vi "THz AcqPan.vi"(8 "error in (no error)":errorcluster caption="entrée d'erreur (pas d'erreur)", 11 "SR830.lvclass":refnum<class "SR830.lvclass">) -> (0 "error out":errorcluster caption="sortie d'erreur", 3 "SR830.lvclass Out":refnum<class "SR830.lvclass">)   [LabVIEW 2012, in "SR830.lvclass"]
uses:
  SR830.lvclass
  BaseDevice/Accessor/GetClassEvent.vi
panel:
  in  "On/Off Delay(ms)":dbl min=0.0 max=10000.0 step=1.0
  in  "Shutter":bool
  out "Sensitivity":u16(ring)=1 items=["2 nV/fA", "5 nV/fA", "10 nV/fA", "20 nV/fA", "50 nV/fA", "100 nV/fA", "200 nV/fA", "500 nV/fA", "1 µV/pA", "2 µV/pA", "5 µV/pA", "10 µV/pA", "20 µV/pA", "50 µV/pA", "100µV/pA", "200 µV/pA", "500µV/pA", "1 mV/nA", "2 mV/nA", "5 mV/nA", "10 mV/nA", "20 mV/nA", "50 mV/nA", "100 mV/nA", "200 mV/nA", "500 mV/nA", "1 V/uA"]
  in  "Acq":bool
  out "Phase":dbl=1000.0 caption="Phase (°)" min=0.0 step=0.1 format="%#_5f"
  out "MAG":dbl=1000.0 caption="MAG (V)" min=0.0 step=0.1 format="%^#_6e"
  out "UNLCK":bool caption="SpexMov"
  out "X":dbl=1000.0 caption="X (V)" min=0.0 step=0.1 format="%^#_6e"
  in  "Stop":bool
  out "Init Program":bool
  out "OVLD":bool caption="SpexMov"
  in  "Update":bool caption="stopSpectro"
  out "Y":dbl=1000.0 caption="Y (V)" min=0.0 step=0.1 format="%^#_6e"
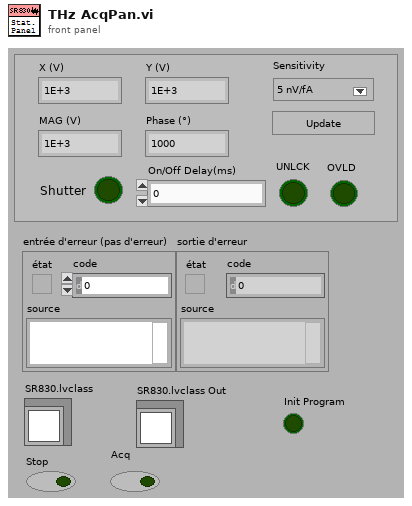
[diagram p1: front panel]
types:
  T1 = enum8{"Enabled", "Disabled", "Disabled and Grayed Out"}
  T2 = enum16{"Phase Shift", "Reference Source", "Reference Frequency", "Reference Trigger", "Detection Harmonic", "Sine Amplitude", "Input Configuration", "Input Shield", "Input Coupling", "Input Line Notch Filter", "Sensitivity", "Dynamic Reserve", "Time Constant", "Low Pass Filter", "Sync Filter", "Expand X", "Expand Y", "Expand R", "All"}
  T3 = cluster{"Phase Shift (°)":dbl, "Reference Source":u16, "Frequency (Hz)":dbl, "Reference Trigger":u16, "Harmonic":i32, "Sine Amplitude (V)":dbl, "Input Configuration":u16, "Input Shield":u16, "Input Coupling":u16, "Input Notch Filters":cluster{"1xLineFilter":bool, "2xLineFilter":bool}, "Sensitivity":u16, "Dynamic Reserve":u16, "Time Constant":u16, "Low Pass Filter":u16, "Sync Filter":bool, "Expand X":cluster{"Offset (%)":dbl, "Expand":u16}, "Expand Y":cluster{"Offset (%)":dbl, "Expand":u16}, "Expand R":cluster{"Offset (%)":dbl, "Expand":u16}}
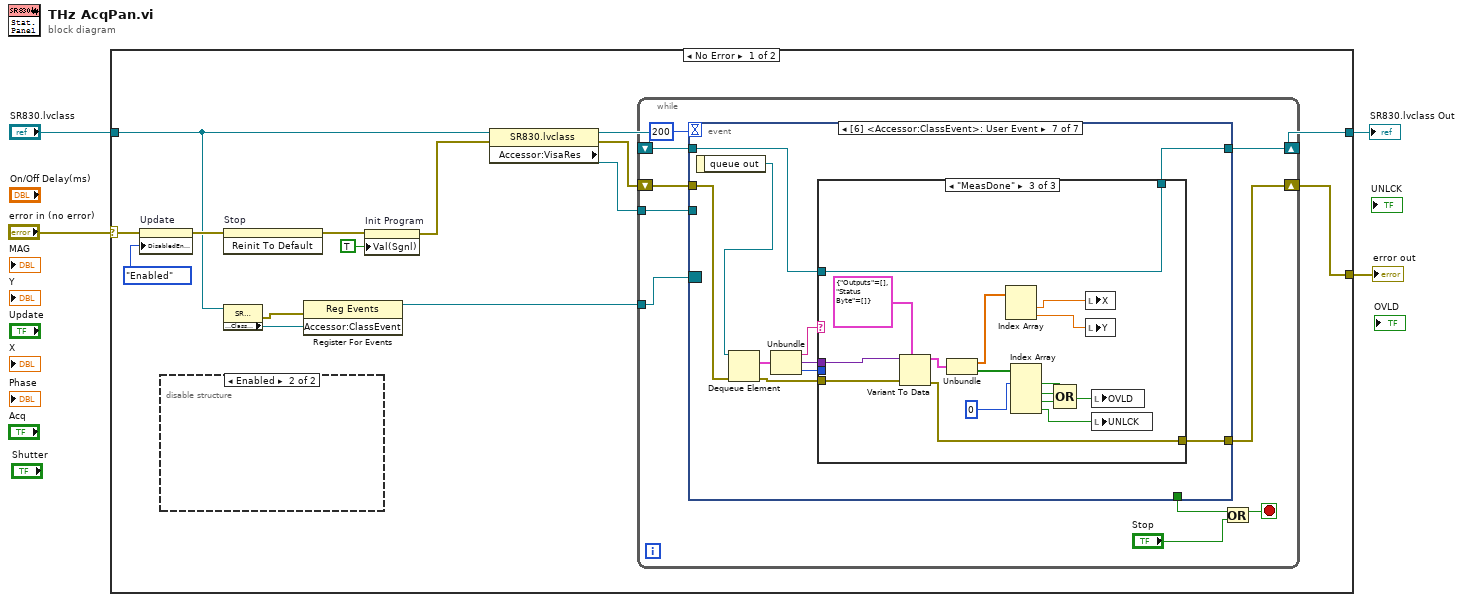
[diagram p0: block diagram]
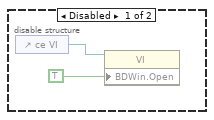
[diagram p2: hidden frame]
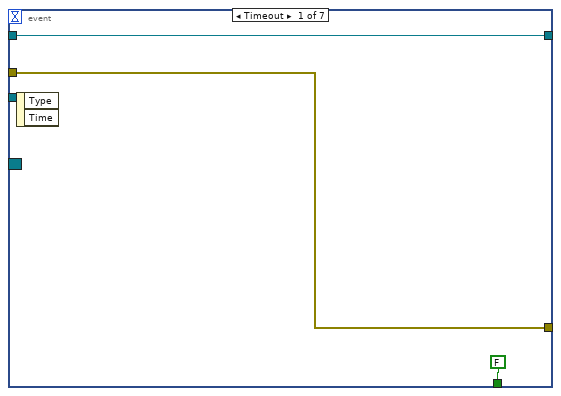
[diagram p3: hidden frame]
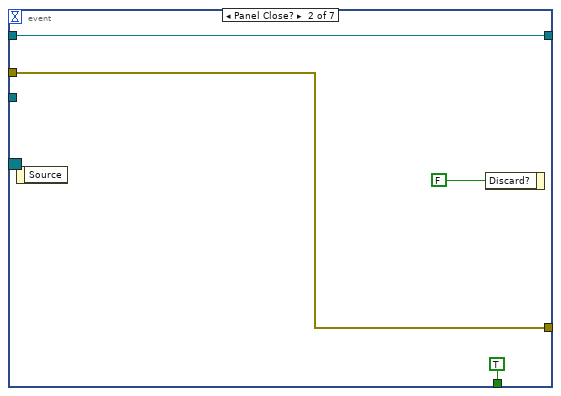
[diagram p4: hidden frame]
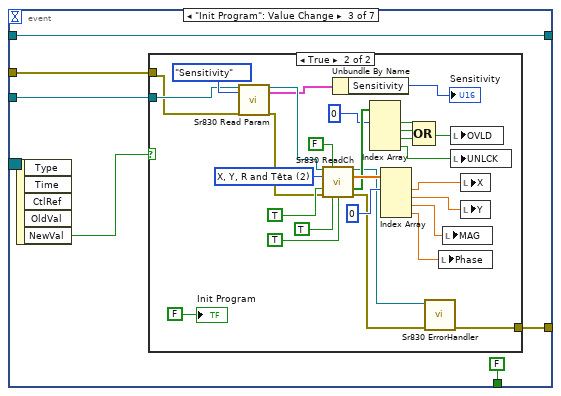
[diagram p5: hidden frame]
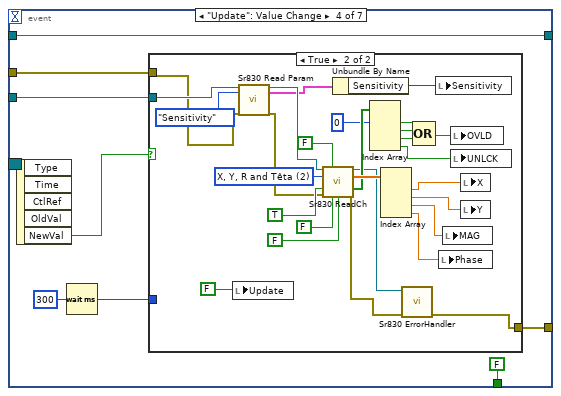
[diagram p7: hidden frame]
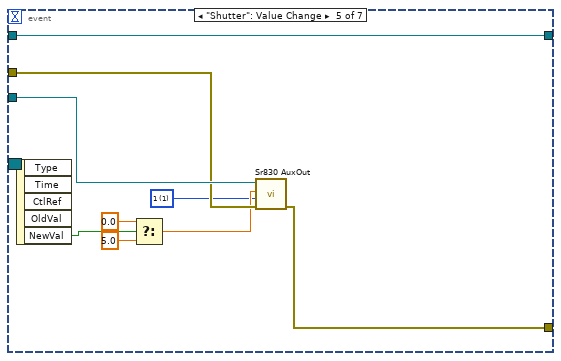
[diagram p9: hidden frame]
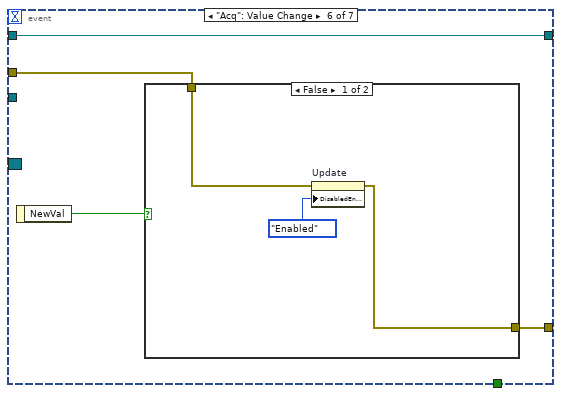
[diagram p10: hidden frame]
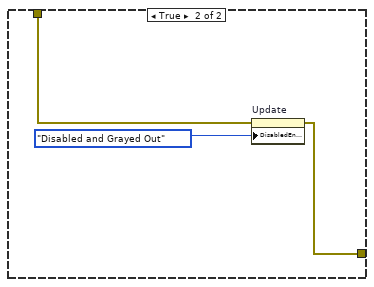
[diagram p11: hidden frame]
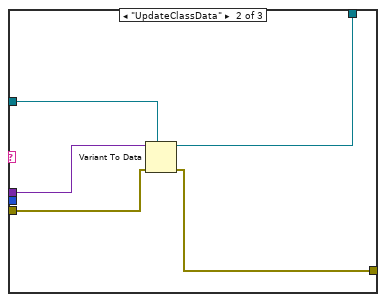
[diagram p13: hidden frame]
diagram:
  n1 = case shown="No Error" "error in (no error)" {
    selector: "error in (no error)" -> [w11 w165]
    tunnel: [w5 w165] -> w3
    tunnel: "SR830.lvclass" -> [w7 w164]
    tunnel: [w17 w164] -> w1
    frame No Error {
      n2 = property on="Update" class="Bool (strict)"(error in=w11, "DisabledEnum"=T1."Enabled" ("Désactivé")) -> (error out=w8:errorcluster)  [unwired: 1 in, 1 out]
      n3 = disable-structure shown="Enabled" {
        frame Disabled {
          n4 = control-ref of="ce VI"() -> (w21:refnum<vi>)
          n5 = property class="VI"(reference=w21, "BDWin.Open"=TRUE ("Fenêtre du diagramme : ouverte")) -> ()  [unwired: 1 in, 2 out]
        }
        frame Enabled {
        }
      }
      n6 = invoke on="Stop" class="Bool (strict)" method="Reinit To Default"(error in=w8) -> (error out=w16:errorcluster)  [unwired: 2 in, 2 out]
      n7 = property class="SR830.lvclass"(reference=w7) -> (error out=w9:errorcluster, "Accessor:ClassEvent"=w10:refnum<user-event>)  [unwired: 1 in, 1 out]
      n8 = register-events(error in=w9, w10) -> (reference out=w6:refnum<event-registration>)  [unwired: 1 in, 1 out]
      n9 = property on="Init Program" class="Bool (strict)"(error in=w16, "Val(Sgnl)"=TRUE ("Valeur (Signalisation)")) -> (error out=w15:errorcluster)  [unwired: 1 in, 1 out]
      n10 = property class="SR830.lvclass"(reference=w7, error in=w15) -> (reference out=w19:refnum<class "SR830.lvclass">, error out=w13:errorcluster, "Accessor:VisaRes"=w14:refnum<visa-resource-name>)
      n11 = while {
        shift-right: [w29] -> w5
        shift-left: w13 -> [w30]
        tunnel: w14 -> [w26]
        shift-right: [w25] -> w17
        shift-left: w19 -> [w28]
        tunnel: w6 -> [w22]
        stop <- w24 stop-if-true
        n12 = event shown="[6] <Accessor:ClassEvent>: User Event" {
          selector: w22 -> [_ _ _ _ _ _ _]
          dyn-events: _ -> [_ _ _ _ _ _ _]
          timeout: 200 -> [_ _ _ _ _ _ _]
          tunnel: w30 -> [w32 w36 w42 w80 w118 w124 w138]
          tunnel: [w32 w36 w41 w79 w117 w122 w131] -> w29
          tunnel: w28 -> [w33 w35 w40 w78 w119 w121 w134]
          tunnel: [FALSE TRUE FALSE FALSE _ _ _] -> w27
          tunnel: [w33 w35 w40 w78 w119 w121 w133] -> w25
          tunnel: w26 -> [_ _ w43 w81 w120 _ _]
          event Timeout {
            n13 = event-data() -> ()  [unwired: 1 in, 2 out]
          }
          event Panel Close? {
            n14 = event-data() -> ()  [unwired: 1 in, 1 out]
            n15 = event-data("Discard?"=FALSE ("Rejeter ?")) -> ()  [unwired: 1 in, 1 out]
          }
          event "Init Program": Value Change {
            n16 = event-data() -> ("NewVal"=w44:bool)  [unwired: 1 in, 4 out]
            n17 = case shown="True" w44 {
              tunnel: w43 -> [_ w58]
              tunnel: w42 -> [w45 w50]
              tunnel: [w45 w48] -> w41
              frame False {
              }
              frame True {
                w66 = u16 2 items=["X and Y", "R and Têta", "X, Y, R and Têta"] ("Channels")
                n18 = call <userlib>:"Sr830 Read Param.vi"("Ressource VISA"=w58, "Énum"=T2."Sensitivity", "error in (no error)"=w50) -> ("Ressource VISA Out"=w57:refnum<visa-resource-name>, "LockInPar"=w56:T3, "error out"=w49:errorcluster)  [unwired: 13 in, 1 out]
                n19 = call <userlib>:"Sr830 ReadCh.vi"("VISA Rsrc"=w57, "Autoscale"=FALSE, "Channels"=w66, "Check Status"=TRUE, "error in (no error)"=w49, "Ask Correction"=TRUE, "Show Warning"=TRUE) -> ("Ressource VISA Out"=w47:refnum<visa-resource-name>, "Outputs"=w73:dbl[], "Status Byte"=w72:bool[], "error out"=w46:errorcluster)  [unwired: 3 in, 2 out]
                n20 = Unbundle By Name(w56) -> ("Sensitivity"=→"Sensitivity":u16)
                n21 = Index Array(array=w72, index #1=0 ("indice")) -> (element #1=w63:bool, element #2=w62:bool, element #3=w61:bool, element #4=w64:bool)  [unwired: 3 in]
                n22 = Index Array(array=w73, index #1=0 ("indice")) -> (element #1=w71:dbl, element #2=w70:dbl, element #3=w69:dbl, element #4=w68:dbl)  [unwired: 3 in]
                n23 = Compound Arithmetic op=OR(w63, w62, w61) -> (w60:bool)
                n24 = call <userlib>:"Sr830 ErrorHandler.vi"("error in (no error)"=w46, "VisaRes"=w47) -> ("error out"=w48:errorcluster)  [unwired: 8 in, 1 out]
                n25 = local write "Phase"(w68) -> ()
                n26 = local write "MAG"(w69) -> ()
                n27 = local write "OVLD"(w60) -> ()
                n28 = local write "UNLCK"(w64) -> ()
                n29 = local write "X"(w71) -> ()
                n30 = local write "Y"(w70) -> ()
                "Init Program" <- FALSE
              }
            }
          }
          event "Update": Value Change {
            n31 = event-data() -> ("NewVal"=w82:bool)  [unwired: 1 in, 4 out]
            n32 = Wait (ms)(milliseconds to wait=u32 300 ("attente (ms)")) -> (millisecond timer value=w75:u32)
            n33 = case shown="True" w82 {
              tunnel: w81 -> [_ w96]
              tunnel: w80 -> [w83 w90]
              tunnel: [w83 w86] -> w79
              tunnel: w75 -> [_ _]
              frame False {
              }
              frame True {
                w104 = u16 2 items=["X and Y", "R and Têta", "X, Y, R and Têta"] ("Channels")
                n34 = local write "Update"(FALSE) -> ()
                n35 = call <userlib>:"Sr830 Read Param.vi"("Ressource VISA"=w96, "Énum"=T2."Sensitivity", "error in (no error)"=w90) -> ("Ressource VISA Out"=w95:refnum<visa-resource-name>, "LockInPar"=w94:T3, "error out"=w89:errorcluster)  [unwired: 13 in, 1 out]
                n36 = call <userlib>:"Sr830 ReadCh.vi"("VISA Rsrc"=w95, "Autoscale"=FALSE, "Channels"=w104, "Check Status"=TRUE, "error in (no error)"=w89, "Ask Correction"=FALSE, "Show Warning"=FALSE) -> ("Ressource VISA Out"=w85:refnum<visa-resource-name>, "Outputs"=w111:dbl[], "Status Byte"=w110:bool[], "error out"=w84:errorcluster)  [unwired: 3 in, 2 out]
                n37 = Unbundle By Name(w94) -> ("Sensitivity"=w93:u16)
                n38 = Index Array(array=w110, index #1=0 ("indice")) -> (element #1=w101:bool, element #2=w100:bool, element #3=w99:bool, element #4=w102:bool)  [unwired: 3 in]
                n39 = Index Array(array=w111) -> (element #1=w109:dbl, element #2=w108:dbl, element #3=w107:dbl, element #4=w106:dbl)  [unwired: 4 in]
                n40 = call <userlib>:"Sr830 ErrorHandler.vi"("error in (no error)"=w84, "VisaRes"=w85) -> ("error out"=w86:errorcluster)  [unwired: 8 in, 1 out]
                n41 = Compound Arithmetic op=OR(w101, w100, w99) -> (w98:bool)
                n42 = local write "Sensitivity"(w93) -> ()
                n43 = local write "Phase"(w106) -> ()
                n44 = local write "MAG"(w107) -> ()
                n45 = local write "OVLD"(w98) -> ()
                n46 = local write "UNLCK"(w102) -> ()
                n47 = local write "X"(w109) -> ()
                n48 = local write "Y"(w108) -> ()
              }
            }
          }
          event "Shutter": Value Change {
            w112 = u16 1 items=["1"=1, "2"=2, "3"=3, "4"=4] ("AuxOut Ch")
            n49 = event-data() -> ("NewVal"=w116:bool)  [unwired: 1 in, 4 out]
            n50 = Select(t=0.0, s=w116, f=5.0) -> (s? t:f=w113:dbl)
            n51 = call <userlib>:"Sr830 AuxOut.vi"("error in"=w118, "AuxOut Ch"=w112, "Voltage"=w113, "Ressource VISA"=w120) -> ("error out"=w117:errorcluster)  [unwired: 1 in, 2 out]
          }
          event "Acq": Value Change {
            n52 = event-data() -> ("NewVal"=w123:bool)  [unwired: 1 in]
            n53 = case shown="False" w123 {
              tunnel: w124 -> [w126 w129]
              tunnel: [w125 w128] -> w122
              frame False {
                n54 = property on="Update" class="Bool (strict)"(error in=w126, "DisabledEnum"=T1."Enabled" ("Désactivé")) -> (error out=w125:errorcluster)  [unwired: 1 in, 1 out]
              }
              frame True {
                n55 = property on="Update" class="Bool (strict)"(error in=w129, "DisabledEnum"=T1."Disabled and Grayed Out" ("Désactivé")) -> (error out=w128:errorcluster)  [unwired: 1 in, 1 out]
              }
            }
          }
          event User Event {
            n56 = event-data() -> ("queue out"=w139:refnum<queue>)  [unwired: 1 in]
            n57 = Dequeue Element(queue=w139, error in (no error)=w138) -> (element=w140:cluster{"Message":string, "Data":variant, i32}, error out=w132:errorcluster)  [unwired: 1 in, 2 out]
            n58 = Unbundle(w140) -> ("Message"=w137:string, "Data"=w136:variant, w135:i32)
            n59 = case shown="\"MeasDone\"" w137 {
              tunnel: w136 -> [_ w145 w162]
              tunnel: w135 -> [_ _ _]
              tunnel: w134 -> [w142 w147 w163]
              tunnel: [w142 w146 w163] -> w133
              tunnel: w132 -> [w141 w144 w160]
              tunnel: [w141 w143 w159] -> w131
              frame Default {
              }
              frame "UpdateClassData" {
                n60 = Variant To Data(error in=w144, type=w147, Variant=w145) -> (data=w146:refnum<class "SR830.lvclass">, error out=w143:errorcluster)
              }
              frame "MeasDone" {
                n61 = Variant To Data(error in=w160, type=cluster{"Outputs":dbl[], "Status Byte":bool[]} {"Outputs"=[], "Status Byte"=[]} ("cluster de sortie"), Variant=w162) -> (data=w156:cluster{"Outputs":dbl[], "Status Byte":bool[]}, error out=w159:errorcluster)
                n62 = Unbundle(w156) -> ("Outputs"=w155:dbl[], "Status Byte"=w149:bool[])
                n63 = Index Array(array=w155) -> (element #1=w158:dbl, element #2=w157:dbl)  [unwired: 2 in]
                n64 = Index Array(array=w149, index #1=0 ("indice")) -> (element #1=w153:bool, element #2=w152:bool, element #3=w151:bool, element #4=w154:bool)  [unwired: 3 in]
                n65 = Compound Arithmetic op=OR(w153, w152, w151) -> (w150:bool)
                n66 = local write "X"(w158) -> ()
                n67 = local write "Y"(w157) -> ()
                n68 = local write "OVLD"(w150) -> ()
                n69 = local write "UNLCK"(w154) -> ()
              }
            }
          }
        }
        n70 = Or(x=w27, y="Stop") -> (x .or. y?=w24:bool)
      }
    }
    frame Error {
    }
  }
  "error out" <- w3
  "SR830.lvclass Out" <- w1
